vi "FIlterResponseTest.vi"() -> ()   [LabVIEW 2014]
uses:
  <instrlib>/Agilent 33XXX Series/Agilent 33XXX Series.lvlib
  <instrlib>/Agilent DSO1000 Series/Agilent DSO1000 Series.lvlib
panel:
  out "Max Power Drop":ext
  out "Result":string
  out "Done":bool
  out "Slide":ext(slide) scale=0.0..100.0 scale format="%#.0g"
  out "Fc Lower Limit":ext
  out "Fc Upper Limit":ext
  out "In Range?":bool
  out "Fc":ext
  out "Ripple Test":bool
  out "Power Drop dB":ext format="%#.6g"
  out "Voltage Out":ext
  out "Voltage In":ext
  out "Frequency":ext caption="Current Freq."
  out "Gain dB":ext
  in  "ResistorUnits":i32(ring) items=["ohm", "Kohm "]
  in  "CapUnits 2":u16(ring) items=["uF", "nF", "pF"]
  in  "C":ext
  in  "R":ext
  # "Filter Response Test for Fc and Ripple"
  # "Running Test Results"
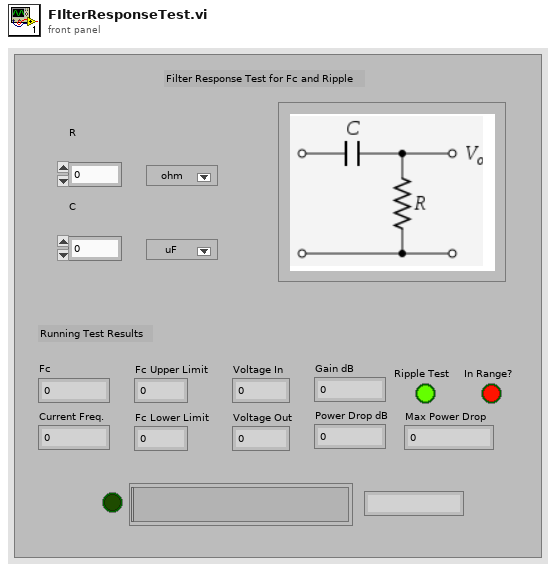
[diagram p1: front panel]
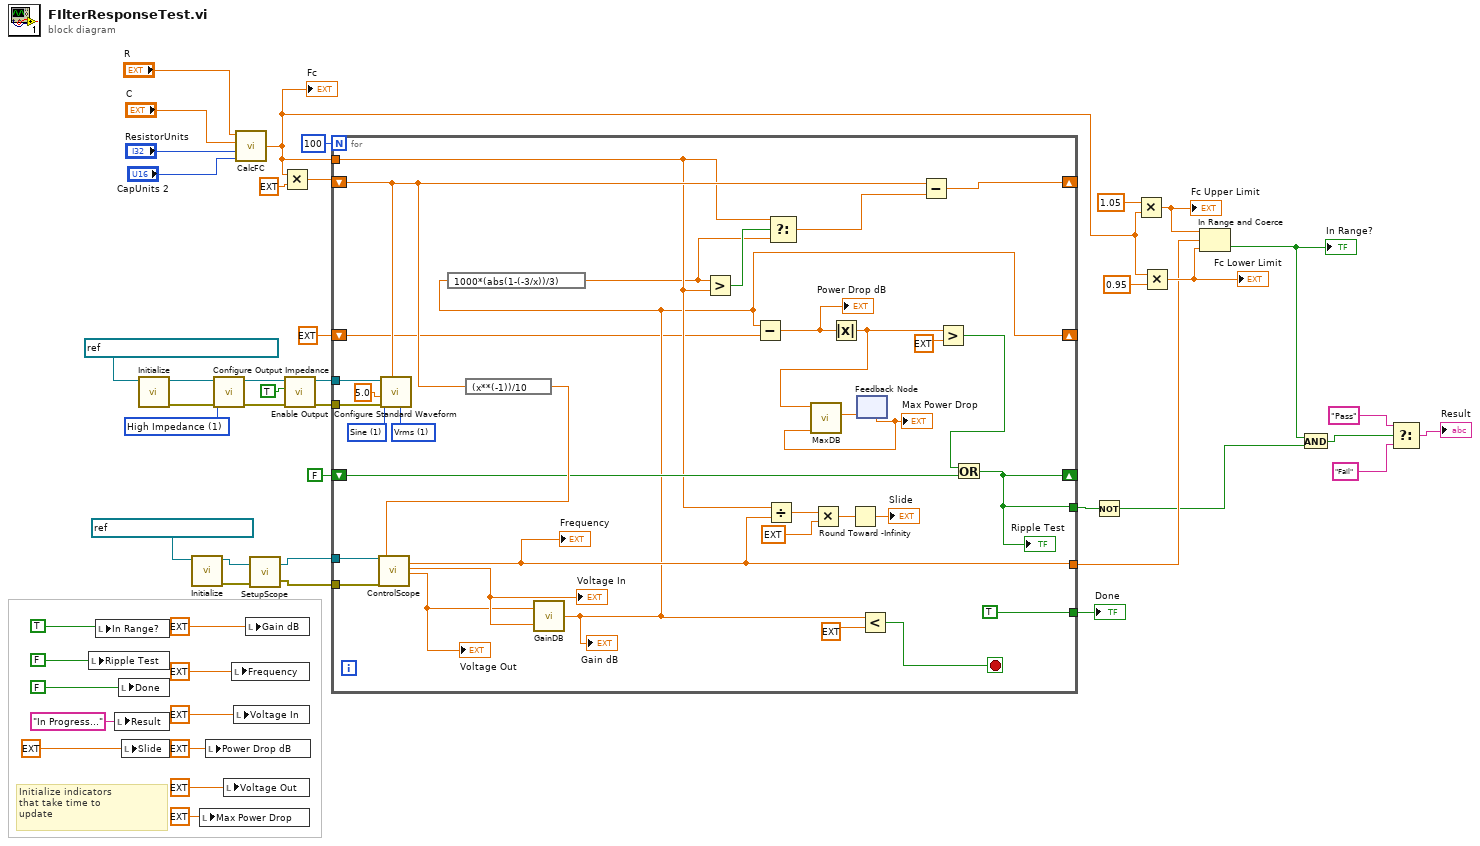
[diagram p0: block diagram]
diagram:
  w45 = u16 1 items=["50 Ohms", "High Impedance", "User Defined"] ("Impedance (0: 50 Ohms)")
  # "Initialize indicators\nthat take time to\nupdate"
  n1 = local write "Ripple Test"(FALSE ("Ripple Test")) -> ()
  n2 = local write "In Range?"(TRUE ("Ripple Test")) -> ()
  n3 = local write "Result"("In Progress..." ("Result")) -> ()
  n4 = local write "Done"(FALSE ("Done")) -> ()
  n5 = local write "Slide"(ext 0.0 ("Slide")) -> ()
  n6 = call <instrlib>:"Initialize.vi"("VISA resource name"=refnum<visa-resource-name> "USB0::0x0957::0x1507::MY48000929::INSTR") -> ("error out"=w46:errorcluster, "VISA resource name out"=w47:refnum<visa-resource-name>)  [unwired: 9 in]
  n7 = call <instrlib>:"Initialize.vi"("VISA resource name"=refnum<visa-resource-name> "USB0::0x0957::0x0588::CN49130420::INSTR") -> ("error out"=w29:errorcluster, "VISA resource name out"=w28:refnum<visa-resource-name>)  [unwired: 9 in]
  n8 = local write "Max Power Drop"(ext 0.0 ("Voltage Out")) -> ()
  n9 = local write "Power Drop dB"(ext 0.0 ("Power Drop dB")) -> ()
  n10 = call <instrlib>:"Configure Output Impedance.vi"("error in (no error)"=w46, "Impedance (0: 50 Ohms)"=w45, "VISA resource name"=w47) -> ("error out"=w43:errorcluster, "VISA resource name out"=w44:refnum<visa-resource-name>)  [unwired: 7 in]
  n11 = local write "Voltage Out"(ext 0.0 ("Voltage Out")) -> ()
  n12 = local write "Frequency"(ext 0.0 ("Frequency")) -> ()
  n13 = local write "Voltage In"(ext 0.0 ("Voltage In")) -> ()
  n14 = call "CalcFC.vi"("CapUnits"="CapUnits 2", "ResistorUnits"="ResistorUnits", "C"="C", "R"="R") -> ("Fc"=w20:ext)
  "Fc" <- w20
  n15 = local write "Gain dB"(ext 0.0 ("Gain dB")) -> ()
  n16 = call "SetupScope.vi"("error in (no error)"=w29, "VISA resource name"=w28) -> ("error out"=w31:errorcluster, "VISA resource name out"=w30:refnum<visa-resource-name>)
  n17 = Multiply(x=w20, y=ext 10.0) -> (x*y=w35:ext)
  n18 = call <instrlib>:"Enable Output.vi"("error in (no error)"=w43, "Enable Output  (T: Enable)"=TRUE, "VISA resource name"=w44) -> ("error out"=w40:errorcluster, "VISA resource name out"=w41:refnum<visa-resource-name>)  [unwired: 7 in]
  n19 = for {
    N: 100 -> [_]
    tunnel: w41 -> [w82]
    tunnel: w40 -> [w81]
    shift-right: [w77] -> _
    shift-left: w35 -> [w68]
    tunnel: w31 -> [w73]
    tunnel: w30 -> [w74]
    tunnel: w20 -> [w63]
    shift-right: [w55] -> _
    shift-left: ext 0.0 ("Voltage Out") -> [w54]
    shift-right: [w53] -> _
    shift-left: FALSE -> [w64]
    tunnel: [w57] -> w21
    tunnel: [TRUE ("Done")] -> w19
    tunnel: [w53] -> w10
    stop <- w75 stop-if-true
    w79 = u16 1 items=["Vpp", "Vrms", "dB"] ("Unit (0: Vpp)")
    w80 = u16 1 items=["DC", "Sine", "Square", "Triangle", "Ramp", "Pulse", "Noise", "Sinc", "Negative Ramp", "Exponential Rise", "Exponential Fall", "Cardiac"] ("Waveform Function (1: Sine)")
    n20 = call <instrlib>:"Configure Standard Waveform.vi"("Unit (0: Vpp)"=w79, "Frequency (1000 Hz)"=w68, "error in (no error)"=w81, "Amplitude (1)"=5.0, "Waveform Function (1: Sine)"=w80, "VISA resource name"=w82) -> ()  [unwired: 4 in, 2 out]
    n21 = expression code="(x**(-1))/10"(w68) -> (w72:ext)
    n22 = call "ControlScope.vi"("VISA resource name"=w74, "error in (no error)"=w73, "Timebase (1E-6 s)"=w72) -> ("Frequency"=w57:ext, "Voltage In"=w71:ext, "Voltage Out"=w67:ext)  [unwired: 12 in, 2 out]
    "Frequency" <- w57
    "Voltage In" <- w71
    "Voltage Out" <- w67
    n23 = call "GainDB.vi"("Vin"=w71, "Vout"=w67) -> ("Gain dB"=w55:ext)
    "Gain dB" <- w55
    n24 = expression code="1000*(abs(1-(-3/x))/3)"(w55) -> (w56:ext)
    n25 = Greater?(x=w56, y=w63) -> (0:w70:bool)
    n26 = Subtract(x=w55, y=w54) -> (x-y=w52:ext)
    "Power Drop dB" <- w52
    n27 = Divide(x=w63, y=w57) -> (x/y=w62:ext)
    n28 = Select(t=w63, s=w70, f=w56) -> (s? t:f=w69:ext)
    n29 = Multiply(x=w62, y=ext 100.0) -> (x*y=w60:ext)
    n30 = Absolute Value(x=w52) -> (abs(x)=w51:ext)
    n31 = Round Toward -Infinity(1:w60) -> (0:→"Slide":ext)
    n32 = feedback #1() -> (w49:ext)  [unwired: 1 in]
    "Max Power Drop" <- w49
    n33 = call "MaxDB.vi"("dBCur"=w51, "db Prev"=w49) -> ("Highest dB"=w50:ext)  [unwired: 8 in]
    n34 = feedback-in #1(w50) -> ()
    n35 = Less?(x=w55, y=ext -3.0) -> (x < y?=w75:bool)
    n36 = Subtract(x=w68, y=w69) -> (x-y=w77:ext)
    n37 = Greater?(x=w51, y=ext 1.0) -> (0:w65:bool)
    n38 = Or(x=w65, y=w64) -> (x .or. y?=w53:bool)
    "Ripple Test" <- w53
  }
  "Done" <- w19
  n39 = Not(x=w10) -> (.not. x?=w11:bool)
  n40 = Multiply(x=1.05, y=w20) -> (x*y=w25:ext)
  "Fc Upper Limit" <- w25
  n41 = Multiply(x=w20, y=0.95) -> (x*y=w24:ext)
  "Fc Lower Limit" <- w24
  n42 = In Range and Coerce(upper limit=w25, x=w21, lower limit=w24) -> (In Range?=w12:bool)  [unwired: 1 out]
  "In Range?" <- w12
  n43 = And(x=w12, y=w11) -> (x .and. y?=w13:bool)
  n44 = Select(t="Pass" ("String 2"), s=w13, f="Fail" ("String 2")) -> (s? t:f=→"Result":string)
